vi "Trim Single line Text.vi"(3 "single-line text":string) -> (1 "trimed text":string)   [LabVIEW 2020, in "Communicable State Machine.lvlib"]
uses:
  Communicable State Machine.lvlib
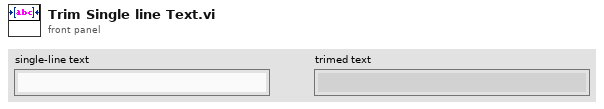
[diagram p1: front panel]
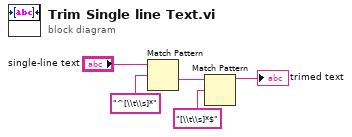
[diagram p0: block diagram]
diagram:
  n1 = Match Pattern(string="single-line text", regular expression="^[\\t\\s]*") -> (after substring=w3:string)  [unwired: 1 in, 3 out]
  n2 = Match Pattern(string=w3, regular expression="[\\t\\s]*$") -> (before substring=→"trimed text":string)  [unwired: 1 in, 3 out]
